vi "actual add tag speed.vi"() -> ()   [LabVIEW 2013, in "tag bus tests.lvlib"]
uses:
  tag bus tests.lvlib
  dictionary/data bus dictionary.lvclass
panel:
  out "data dictionary out":refnum<class "data bus dictionary.lvclass">
  out "error out":errorcluster
  in  "count":i32=5000
  out "time":dbl
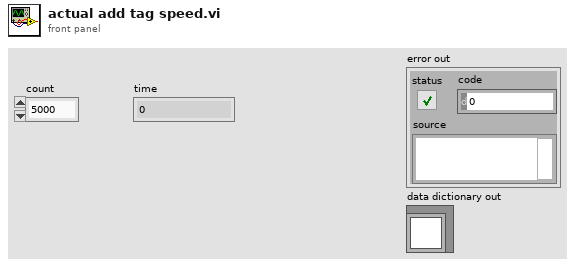
[diagram p1: front panel]
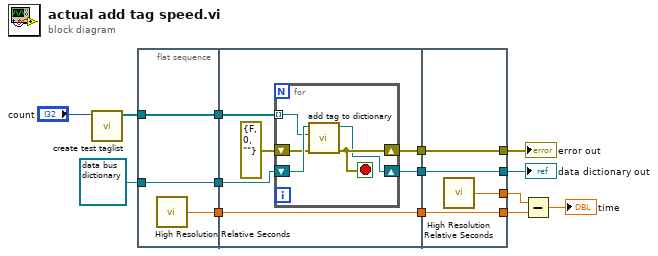
[diagram p0: block diagram]
diagram:
  n1 = call "create test taglist.vi"("count"="count") -> ("tags"=w8:refnum<class "data bus tag description.lvclass">[])  [unwired: 7 in, 3 out]
  n2 = flat-sequence {
    tunnel: [w17] -> w13
    tunnel: [w16] -> w9
    tunnel: w8 -> [w16]
    tunnel: [w15] -> w6
    tunnel: refnum<class "data bus dictionary.lvclass"> refnum ("data dictionary out") -> [w15]
    tunnel: w13 -> [w23]
    tunnel: [w23] -> w12
    tunnel: w9 -> [w21]
    tunnel: w6 -> [w22]
    tunnel: [w19] -> w4
    tunnel: [w18] -> w2
    tunnel: [w32] -> w14
    tunnel: w12 -> [w31]
    tunnel: [w31] -> w11
    tunnel: [w30] -> w3
    tunnel: w4 -> [w30]
    tunnel: [w29] -> w1
    tunnel: w2 -> [w29]
    frame #0 {
      n3 = call <vilib>:"High Resolution Relative Seconds.vi"() -> ("relative seconds"=w17:dbl)
    }
    frame #1 {
      n4 = for {
        shift-right: [w28] -> w19
        shift-left: errorcluster {"status"=FALSE, "code"=0, "source"=""} ("error out") -> [w24]
        shift-right: [w27] -> w18
        shift-left: w22 -> [w26]
        tunnel: w21 -> [w25] mode=indexing
        stop <- w28 stop-if-true
        n5 = call "add tag to dictionary.vi"("error in"=w24, "system tag"=w25, "data dictionary in"=w26) -> ("error out"=w28:errorcluster, "data dictionary out"=w27:refnum<class "data bus dictionary.lvclass">)  [unwired: 7 in]
      }
    }
    frame #2 {
      n6 = call <vilib>:"High Resolution Relative Seconds.vi"() -> ("relative seconds"=w32:dbl)
    }
  }
  n7 = Subtract(x=w14, y=w11) -> (x-y=→"time":dbl)
  "error out" <- w3
  "data dictionary out" <- w1
